vi "Load Config.vi"(8 "error in (no error)":errorcluster, 11 "DAQmxVoltageChannel in":refnum<class "VoltageInChannel.lvclass">) -> (0 "error out":errorcluster, 3 "DAQmxVoltageChannel out":refnum<class "VoltageInChannel.lvclass">)   [LabVIEW 2020, in "VolatusDAQConfig.lvlib" / "VoltageInChannel.lvclass"]
uses:
  VoltageInChannel.lvclass
  C:/dev/lv20CE/relink/lv-volatus/VolatusConfig/VolatusConfigElement/VolatusConfigElement.lvclass
  VolatusConfig/VolatusConfigElement/VolatusConfigElement.lvclass/VolatusConfigElement.ctl
  VoltageInChannel.lvclass/VoltageInChannel.ctl
  VolatusConfig/VolatusConfigElement/Element.vi
  VolatusConfig/VolatusConfigElement/VolatusConfigElement.lvclass
  lv-cdm/CDM-Config/Config Element/Config Element.lvclass
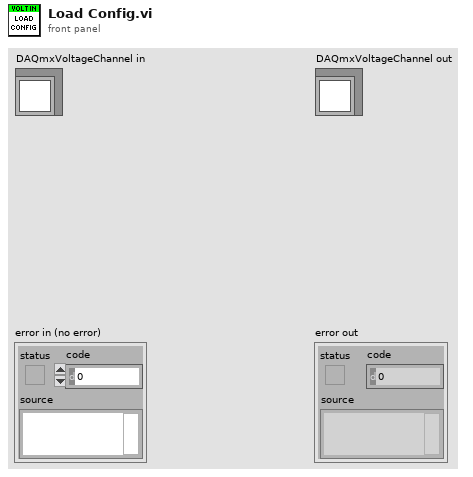
[diagram p1: front panel]
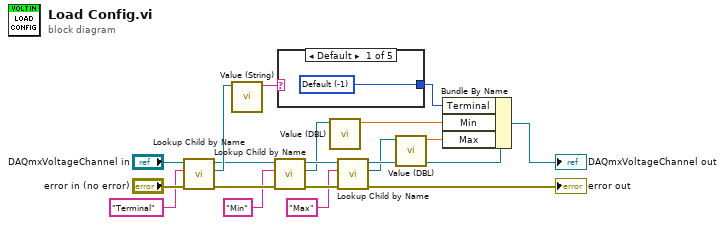
[diagram p0: block diagram]
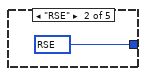
[diagram p2: hidden frame]
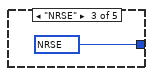
[diagram p3: hidden frame]
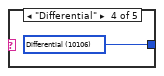
[diagram p4: hidden frame]
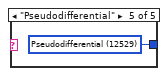
[diagram p5: hidden frame]
diagram:
  n1 = call "Lookup Child by Name.vi"("error in (no error)"="error in (no error)", "Child Name"="Terminal", "VolatusConfigElement in"="DAQmxVoltageChannel in") -> ("error out"=w18:errorcluster, "Child"=w15:refnum<class "Config Element.lvclass">, "VolatusConfigElement out"=w10:refnum<class "VoltageInChannel.lvclass">)  [unwired: 5 in, 1 out]
  n2 = call "Value (String).vi"("Config Element in"=w15) -> ("String Value"=w14:string)  [unwired: 9 in, 1 out]
  n3 = call "Lookup Child by Name.vi"("error in (no error)"=w18, "Child Name"="Min", "VolatusConfigElement in"=w10) -> ("error out"=w11:errorcluster, "Child"=w5:refnum<class "Config Element.lvclass">, "VolatusConfigElement out"=w8:refnum<class "VoltageInChannel.lvclass">)  [unwired: 5 in, 1 out]
  n4 = case shown="Default" w14 {
    tunnel: [w20 w21 w22 w23 w24] -> w13
    frame Default {
      w20 = -1 items=["Default"=-1, "RSE"=10083, "NRSE"=10078, "Differential"=10106, "Pseudodifferential"=12529] ("input terminal configuration")
    }
    frame "RSE" {
      w21 = 10083 items=["Default"=-1, "RSE"=10083, "NRSE"=10078, "Differential"=10106, "Pseudodifferential"=12529] ("input terminal configuration")
    }
    frame "NRSE" {
      w22 = 10078 items=["Default"=-1, "RSE"=10083, "NRSE"=10078, "Differential"=10106, "Pseudodifferential"=12529] ("input terminal configuration")
    }
    frame "Differential" {
      w23 = 10106 items=["Default"=-1, "RSE"=10083, "NRSE"=10078, "Differential"=10106, "Pseudodifferential"=12529] ("input terminal configuration")
    }
    frame "Pseudodifferential" {
      w24 = 12529 items=["Default"=-1, "RSE"=10083, "NRSE"=10078, "Differential"=10106, "Pseudodifferential"=12529] ("input terminal configuration")
    }
  }
  n5 = call "Value (DBL).vi"("Config Element in"=w5) -> ("DBL Value"=w4:dbl)  [unwired: 9 in, 1 out]
  n6 = call "Lookup Child by Name.vi"("error in (no error)"=w11, "Child Name"="Max", "VolatusConfigElement in"=w8) -> ("error out"=→"error out":errorcluster, "Child"=w3:refnum<class "Config Element.lvclass">, "VolatusConfigElement out"=w7:refnum<class "VoltageInChannel.lvclass">)  [unwired: 5 in, 1 out]
  n7 = call "Value (DBL).vi"("Config Element in"=w3) -> ("DBL Value"=w2:dbl)  [unwired: 9 in, 1 out]
  n8 = Bundle By Name(cluster=w7, "Terminal"=w13, "Min"=w4, "Max"=w2) -> (→"DAQmxVoltageChannel out":refnum<class "VoltageInChannel.lvclass">)
